vi "WebView2_EscapePath.vi"(11 "Path":path) -> (3 "File Path":string)   [LabVIEW 2020, in "WebView2-Viewer.lvlib"]
uses:
  WebView2-Viewer.lvlib
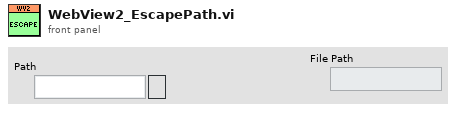
[diagram p1: front panel]
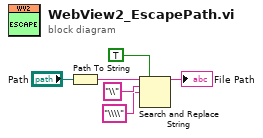
[diagram p0: block diagram]
diagram:
  n1 = Path To String(path="Path") -> (string=w5:string)
  n2 = Search and Replace String(replace all?=TRUE ("replace all? (F)"), input string=w5, search string="\\", replace string="\\\\" ("replace string (\"\")")) -> (result string=→"File Path":string)  [unwired: 4 in, 3 out]
